vi "Measure Voltage.vi"(8 "error in (no error)":errorcluster, 11 "N5745A in":refnum<class "5745A.lvclass">) -> (0 "error out":errorcluster, 2 "Voltage":dbl format="%.6f", 3 "N5745A out":refnum<class "5745A.lvclass">)   [LabVIEW 2018, in "5745A.lvlib" / "5745A.lvclass"]
doc: "This Override method outputs voltage measurement from N5745a instrument."
uses:
  5745A.lvclass
  builds/Power_Supply.lvlibp/Power Supply.lvclass
  C:/Users/Ron.Dexter.LUMINARTECH/Desktop/builds/Power_Supply.lvlibp/Power Supply.lvclass
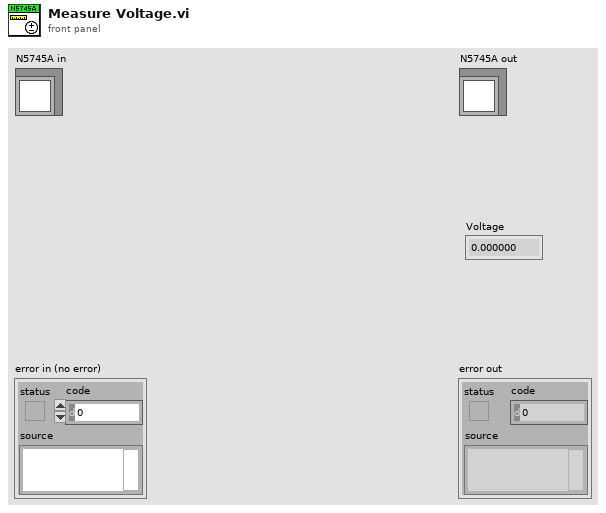
[diagram p1: front panel]
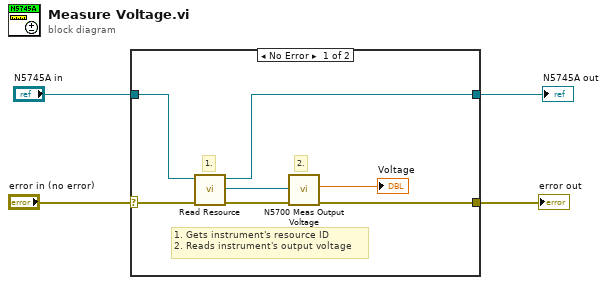
[diagram p0: block diagram]
diagram:
  n1 = case shown="No Error" "error in (no error)" {
    selector: "error in (no error)" -> [w10 w12]
    tunnel: [w5 w13] -> w2
    tunnel: "N5745A in" -> [w6 w13]
    tunnel: [w7 w12] -> w1
    frame No Error {
      # "1. Gets instrument's resource ID\n2. Reads instrument's output voltage"
      # "2."
      # "1."
      n2 = call "Read Resource.vi"("error in"=w10, "Power Supply in"=w6) -> ("error out"=w8:errorcluster, "Resource"=w9:refnum<visa-resource-name>, "Power Supply out"=w5:refnum<class "5745A.lvclass">)  [unwired: 7 in]
      n3 = call <instrlib>:"N5700 Meas Output Voltage.vi"("error"=w8, "VISA"=w9) -> ("error out"=w7:errorcluster, "Output Voltage"=→"Voltage":dbl)  [unwired: 4 in, 1 out]
    }
    frame Error {
    }
  }
  "error out" <- w1
  "N5745A out" <- w2
